vi "Untitled 3 (Message builder).vi"(9 "Array":dbl[](array[numeric]), 10 "String":string, 11 "msg in":string) -> (3 "msg out":string)   [LabVIEW 2016]
uses:
  builds/UnicornMain/UnicornRIO1/ROS for LabVIEW/home/lvuser/natinst/bin/user.lib/ROS for LabVIEW Software/ROS/MessageBuilding/std_msgs/subs/stringScalar.vi
  builds/UnicornMain/UnicornRIO1/ROS for LabVIEW/home/lvuser/natinst/bin/user.lib/ROS for LabVIEW Software/ROS/MessageBuilding/std_msgs/subs/float32Array.vi
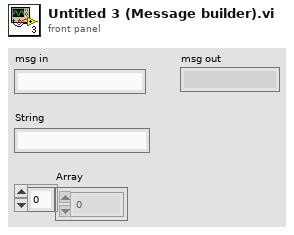
[diagram p1: front panel]
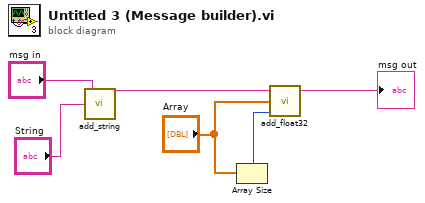
[diagram p0: block diagram]
diagram:
  n1 = call-poly "add_string.vi"("String"="String", "msg in"="msg in") -> ("msg out"=w4:string)  [unwired: 3 in]
  n2 = Array Size(array="Array") -> (size(s)=w3:i32)
  n3 = call-poly "add_float32.vi"("Array Length"=w3, "Array"="Array", "msg in"=w4) -> ("msg out"=→"msg out":string)  [unwired: 2 in]
